vi "Global 1.vi"() -> ()   [LabVIEW 2019]
uses:
  TPC-Enum.ctl
panel:
  in  "Test request":string
  out "Main Loop Status":string
  out "TCP loop status":T1
  out "Labview response":string
  out "Received request":string
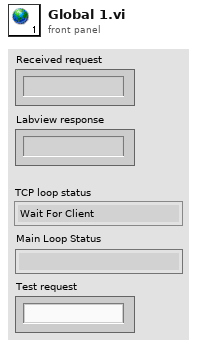
[diagram p1: front panel]
types:
  T1 = typedef "TPC-Enum.ctl" = enum16{"Wait For Client", "Check Client", "Listen"}
diagram:
